vi "Build Numbered String Map.vi"(10 "Strings":string[](array[string])) -> (2 "Map":map{string, string}(c390))   [LabVIEW 2022 SP3]
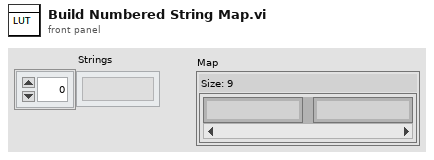
[diagram p1: front panel]
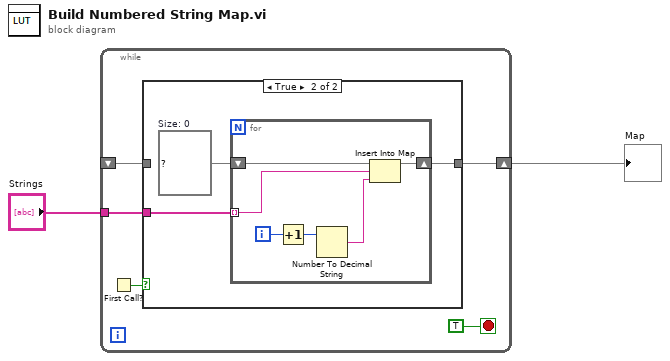
[diagram p0: block diagram]
diagram:
  n1 = while {
    tunnel: "Strings" -> [w7]
    shift-right: [w4] -> w1
    shift-left: _ -> [w5]
    stop <- TRUE stop-if-true
    n2 = First Call?() -> (First Call?: T/F=w6:bool)
    n3 = case shown="True" w6 {
      tunnel: w7 -> [_ w11]
      tunnel: w5 -> [w8 _]
      tunnel: [w8 w10] -> w4
      frame False {
      }
      frame True {
        w9 = map{string, string} {}  # Size: 0
        n4 = for {
          tunnel: w11 -> [w14] mode=indexing
          shift-right: [w12] -> w10
          shift-left: w9 -> [w15]
          i -> [w17]
          n5 = Increment(x=w17) -> (x+1=w16:i32)
          n6 = Number To Decimal String(number=w16) -> (decimal integer string=w13:string)  [unwired: 1 in]
          n7 = Insert Into Map(map in=w15, key=w14, value=w13) -> (map out=w12:map{string, string})  [unwired: 2 out]
        }
      }
    }
  }
  "Map" <- w1
